vi "Lift.vi"(1 "Level":i16, 2 "Manual":dbl) -> (0 "At Level":bool)   [LabVIEW 2014]
uses:
  <vilib>/Rock Robotics/WPI/Solenoid/WPI_SolenoidValue.ctl
  <vilib>/Rock Robotics/Network Tables/SD Write Number.vi
  <vilib>/Rock Robotics/WPI/Solenoid/WPI_SolenoidSetEnum.vi
  <vilib>/Rock Robotics/Network Tables/SD Write Boolean.vi
  <vilib>/addons/control/pid/pid.llb/PID (DBL).vi
  <vilib>/addons/control/pid/NI_PID_pid.lvlib
panel:
  in  "high speeds":cluster{"output high":dbl, "output low":dbl}={"output high"=1.0, "output low"=-0.7}
  in  "low speeds":cluster{"output high":dbl, "output low":dbl}={"output high"=0.8, "output low"=-0.6}
  out "Motor Output":dbl(graph)
  in  "Tote height":dbl=12.25
  in  "Lift constant":dbl=9.5
  in  "Coopertition":dbl=15.0
  in  "Container":dbl=0.25 format="%#_13g"
  in  "Transport":dbl=12.0
  in  "Under tote":dbl=4.0
  out "Lift Current":dbl(knob) scale=0.0..30.0
  out "lim":bool
  in  "PID gains":T1={"proportional gain (Kc)"=0.55, "integral time (Ti, min)"=0.0, "derivative time (Td, min)"=0.001}
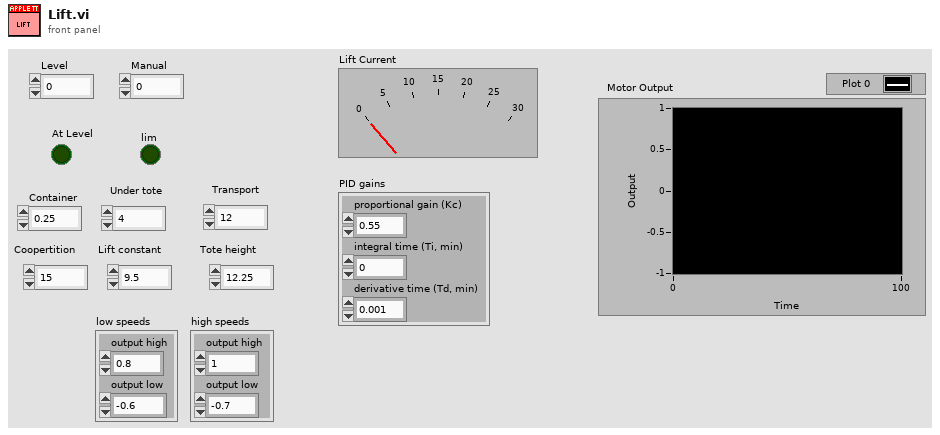
[diagram p1: front panel]
types:
  T1 = cluster{"proportional gain (Kc)":dbl, "integral time (Ti, min)":dbl, "derivative time (Td, min)":dbl}
  T2 = typedef "WPI_SolenoidValue.ctl" = enum16{"Off", "On", "Forward", "Reverse"}
  T3 = typedef "WPI_DigitalInputDevRef.ctl" = cluster{"DevStatus":errorcluster, "DIO Channel":T4, "Controller":T5}
  T4 = typedef "FPGA_DIOChannel.ctl" = enum8{"DIO 0", "DIO 1", "DIO 2", "DIO 3", "DIO 4", "DIO 5", "DIO 6", "DIO 7", "DIO 8", "DIO 9", "DIO MXP 0", "DIO MXP 1", "DIO MXP 2", "DIO MXP 3", "DIO MXP 4", "DIO MXP 5", "DIO MXP 6", "DIO MXP 7", "DIO MXP 8", "DIO MXP 9", "DIO MXP 10", "DIO MXP 11", "DIO MXP 12", "DIO MXP 13", "DIO MXP 14", "DIO MXP 15", "Invalid"}
  T5 = typedef "FPGA_TypedefDigitalModule.ctl" = enum16{"Controller 1"}
  T6 = typedef "WPI_EncoderDevRef.ctl" = cluster{"DevStatus":errorcluster, "EncoderIndex":T7, "CounterIndex":T8, "DistancePerCount":dbl, "Decoding Type":T9}
  T7 = typedef "FPGA_EncoderIdx.ctl" = enum8{"Enc 0", "Enc 1", "Enc 2", "Enc 3", "Enc 4", "Enc 5", "Enc 6", "Enc 7", "Invalid"}
  T8 = typedef "FPGA_CounterCtrSystemIndex.ctl" = enum8{"Ctr 0", "Ctr 1", "Ctr 2", "Ctr 3", "Ctr 4", "Ctr 5", "Ctr 6", "Ctr 7", "Invalid"}
  T9 = typedef "WPI_EncoderType.ctl" = enum16{"1x", "2x", "4x"}
  T10 = typedef "WPI_SolenoidDevRef.ctl" = cluster{"DevStatus":errorcluster, "Pneumatics Control Module":u8, "Forward Solenoid Channel":T11, "Reverse Solenoid Channel":T11}
  T11 = typedef "WPI_SolenoidChannel.ctl" = enum8{"Solenoid 0", "Solenoid 1", "Solenoid 2", "Solenoid 3", "Solenoid 4", "Solenoid 5", "Solenoid 6", "Solenoid 7", "Invalid"}
  T12 = typedef "WPI_MotorControlDeviceRef.ctl" = cluster{"DeviceStatus":errorcluster, "Type":T13, "PWM":cluster{"Controller":T5, "PWM Channel":T14, "DeadBand":T15}, "CAN":cluster{"Device Number":u8, "Control Mode":T16, "Semaphore":T17, "Max Vout":dbl, "TalonSRX Control Mode":T18}, "Invert":bool, "TransformRef":T19, "InvTransformRef":T19}
  T13 = typedef "WPI_MotorControlType.ctl" = enum16{"PWM", "CAN", "CANTalonSRX"}
  T14 = typedef "FPGA_DIOPWMChannel.ctl" = enum8{"PWM 0", "PWM 1", "PWM 2", "PWM 3", "PWM 4", "PWM 5", "PWM 6", "PWM 7", "PWM 8", "PWM 9", "PWM MXP 0", "PWM MXP 1", "PWM MXP 2", "PWM MXP 3", "PWM MXP 4", "PWM MXP 5", "PWM MXP 6", "PWM MXP 7", "PWM MXP 8", "PWM MXP 9", "Invalid"}
  T15 = typedef "WPI_PWMDeadband.ctl" = cluster{"Name":string, "maxPositivePwm":i32, "minPositivePwm":i32, "centerPwm":i32, "maxNegativePwm":i32, "minNegativePwm":i32, "angularRange":u16}
  T16 = typedef "WPI_CANJaguar_ControlMode.ctl" = enum8{"Percent VBus", "Current", "Speed", "Position", "Voltage"}
  T17 = typedef "Semaphore RefNum" = refnum<k1>
  T18 = typedef "WPI_CANTalonSRX_APIControlMode.ctl" = enum8{"Percent VBus", "Speed", "Position", "Slave", "Unchanged / Invalid"}
  T19 = typedef "WPI_PWMTransform_ConPane.ctl" = refnum<vi>
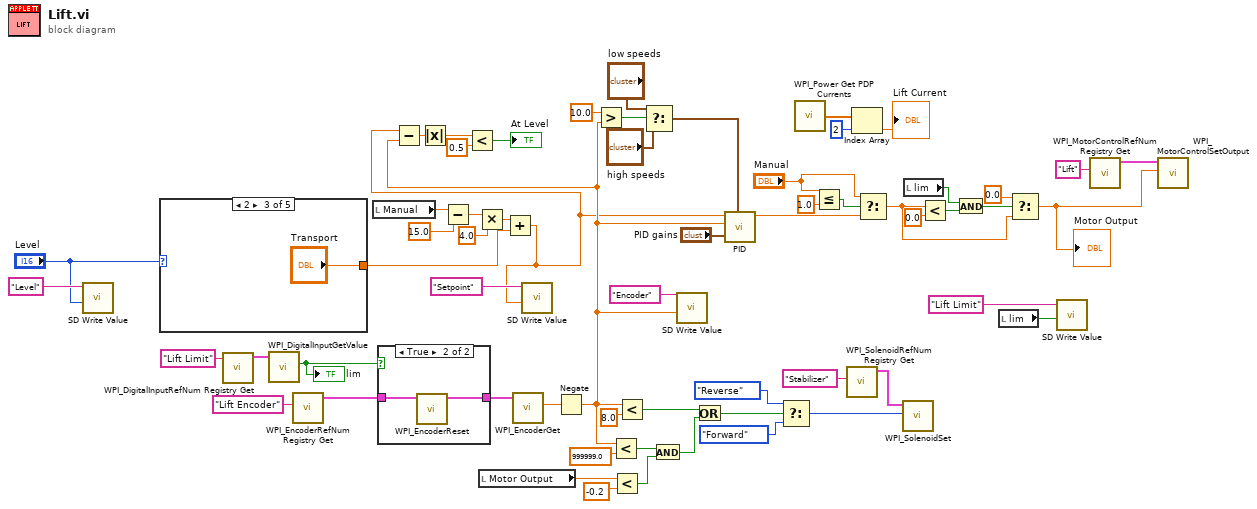
[diagram p0: block diagram]
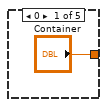
[diagram p2: hidden frame]
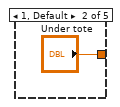
[diagram p3: hidden frame]
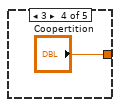
[diagram p4: hidden frame]
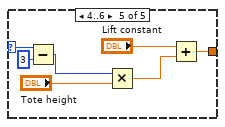
[diagram p5: hidden frame]
diagram:
  n1 = call-poly <vilib>:"SD Write Value.vi"("Numeric"="Level", "Name"="Level") -> ()  [unwired: 8 in, 2 out]
  n2 = case shown="2" "Level" {
    selector: "Level" -> [_ _ _ _ w72]
    tunnel: ["Container" "Under tote" "Transport" "Coopertition" w68] -> w5
    frame 0 {
    }
    frame 1, Default {
    }
    frame 2 {
    }
    frame 3 {
    }
    frame 4..6 {
      n3 = Subtract(x=w72, y=i16 3) -> (x-y=w71:i16)
      n4 = Multiply(x=w71, y="Tote height") -> (x*y=w66:dbl)
      n5 = Add(x="Lift constant", y=w66) -> (x+y=w68:dbl)
    }
  }
  n6 = call <vilib>:"WPI_DigitalInputRefNum Registry Get.vi"("refnum name"="Lift Limit") -> ("DigitalInputDevRef"=w47:T3)  [unwired: 9 in, 1 out]
  n7 = call <vilib>:"WPI_DigitalInputGetValue.vi"("DigitalInputDevRef"=w47) -> ("Value"=w46:bool)  [unwired: 8 in, 2 out]
  "lim" <- w46
  n8 = call <vilib>:"WPI_EncoderRefNum Registry Get.vi"("refnum name"="Lift Encoder") -> ("EncoderDevRef"=w58:T6)  [unwired: 9 in, 1 out]
  n9 = local read "Manual"() -> (w10:dbl)
  n10 = case shown="True" w46 {
    tunnel: w58 -> [w73 w75]
    tunnel: [w73 w74] -> w60
    frame False {
    }
    frame True {
      n11 = call <vilib>:"WPI_EncoderReset.vi"("EncoderDevRef"=w75) -> ("EncoderDevRef"=w74:T6)  [unwired: 1 in, 9 out]
    }
  }
  n12 = Subtract(x=w10, y=15.0) -> (x-y=w8:dbl)
  n13 = Multiply(x=w8, y=4.0) -> (x*y=w6:dbl)
  n14 = local read "Motor Output"() -> (w29:dbl)
  n15 = Add(x=w6, y=w5) -> (x+y=w4:dbl)
  n16 = call <vilib>:"WPI_EncoderGet.vi"("EncoderDevRef"=w60) -> ("Distance"=w57:dbl)  [unwired: 5 in, 5 out]
  n17 = call-poly <vilib>:"SD Write Value.vi"("Numeric"=w4, "Name"="Setpoint") -> ()  [unwired: 8 in, 2 out]
  n18 = Negate(x=w57) -> (-x=w16:dbl)
  n19 = Subtract(x=w4, y=w16) -> (x-y=w56:dbl)
  n20 = Absolute Value(x=w56) -> (abs(x)=w49:dbl)
  n21 = Less?(x=w49, y=0.5) -> (x < y?=→"At Level":bool)
  n22 = Greater?(x=10.0, y=w16) -> (0:w53:bool)
  n23 = Less?(x=w16, y=999999.0) -> (x < y?=w32:bool)
  n24 = Less?(x=w29, y=-0.2) -> (x < y?=w27:bool)
  n25 = Less?(x=w16, y=8.0) -> (x < y?=w34:bool)
  n26 = Select(t="low speeds", s=w53, f="high speeds") -> (s? t:f=w50:cluster{"output high":dbl, "output low":dbl})
  n27 = And(x=w32, y=w27) -> (x .and. y?=w31:bool)
  n28 = call-poly <vilib>:"SD Write Value.vi"("Numeric"=w16, "Name"="Encoder") -> ()  [unwired: 8 in, 2 out]
  n29 = Or(x=w34, y=w31) -> (x .or. y?=w30:bool)
  n30 = call-poly <vilib>:"PID.vi"("output range"=w50, "PID gains"="PID gains", "process variable"=w16, "setpoint"=w4) -> ("output"=w3:dbl)  [unwired: 6 in, 1 out]
  n31 = Select(t=WPI_SolenoidValue."Reverse" ("Value"), s=w30, f=WPI_SolenoidValue."Forward" ("Value")) -> (s? t:f=w24:T2)
  n32 = call <vilib>:"WPI_Power Get PDP Currents.vi"() -> ("all currents (A)"=w38:dbl[])  [unwired: 13 in, 2 out]
  n33 = Less Or Equal?(x="Manual", y=1.0) -> (x <= y?=w13:bool)
  n34 = call <vilib>:"WPI_SolenoidRefNum Registry Get.vi"("refnum name"="Stabilizer") -> ("SolenoidDevRef"=w35:T10)  [unwired: 9 in, 1 out]
  n35 = Index Array(array=w38, index=2) -> (element=→"Lift Current":dbl)
  n36 = Select(t="Manual", s=w13, f=w3) -> (s? t:f=w2:dbl)
  n37 = call-poly <vilib>:"WPI_SolenoidSet.vi"("Value"=w24, "SolenoidDevRef"=w35) -> ()  [unwired: 8 in, 2 out]
  n38 = local read "lim"() -> (w43:bool)
  n39 = Less?(x=w2, y=0.0) -> (x < y?=w44:bool)
  n40 = And(x=w43, y=w44) -> (x .and. y?=w42:bool)
  n41 = local read "lim"() -> (w21:bool)
  n42 = Select(t=0.0, s=w42, f=w2) -> (s? t:f=w1:dbl)
  "Motor Output" <- w1
  n43 = call-poly <vilib>:"SD Write Value.vi"("Boolean"=w21, "Name"="Lift Limit") -> ()  [unwired: 8 in, 2 out]
  n44 = call <vilib>:"WPI_MotorControlRefNum Registry Get.vi"("refnum name"="Lift") -> ("MotorControlDevRef"=w22:T12)  [unwired: 9 in, 1 out]
  n45 = call <vilib>:"WPI_MotorControlSetOutput.vi"("Output"=w1, "MotorControlDevRef"=w22) -> ()  [unwired: 7 in, 3 out]
